vi "Autonomous Independent.vi"() -> ()   [LabVIEW 2018]
doc: "This VI is called when autonomous begins, and will automatically be terminated when autonomous ends. You can carry out timed or sensor driven robot movement independently without needing to return to the caller."
uses:
  <vilib>/Rock Robotics/WPI/Utilities/WPI_GetSetVariantRefNum.vi
  <vilib>/Rock Robotics/Network Tables/NT Read String.vi
  <vilib>/Rock Robotics/Network Tables/NT Write Numeric Array.vi
  <vilib>/Rock Robotics/Network Tables/NT Read Boolean.vi
  <vilib>/Rock Robotics/Network Tables/NT Write Boolean Array.vi
  <vilib>/Rock Robotics/Network Tables/NT Write Boolean.vi
  <vilib>/Rock Robotics/Network Tables/NT Write Number.vi
  <vilib>/Rock Robotics/Network Tables/NT Read Number.vi
  <vilib>/Rock Robotics/Network Tables/NT Read Numeric Array.vi
panel:
  in  "Motor Stall":dbl format="%#_13g"
  out "Current Movement, for debugging":T1 {"Y Joystick Value" scale=1.0..-1.0; "X Joystick Value" scale=-1.0..1.0}
  in  "Array of robot movements":T2(array[cluster])=[{"X Joystick Value"=0.39393939393939403, "Y Joystick Value"=0.0, "Delay (sec)"=1.0, "Movement Name"="turn"}, {"X Joystick Value"=-0.3737373737373737, "Y Joystick Value"=0.0, "Delay (sec)"=1.0, "Movement Name"="turn back"}] {"Y Joystick Value" scale=1.0..-1.0; "X Joystick Value" scale=-1.0..1.0}
  # "Be sure to right-click and choose Data Operations>>Make Current Value default if you want to save the array values with the VI"
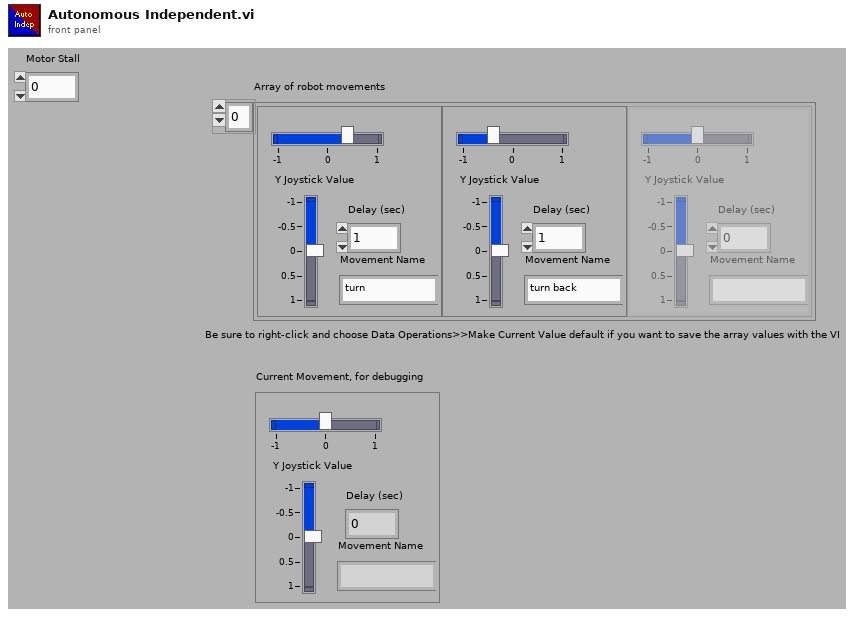
[diagram p1: front panel]
types:
  T1 = cluster{"X Joystick Value":dbl, "Y Joystick Value":dbl, "Delay (sec)":dbl, "Movement Name":string}
  T2 = cluster{"X Joystick Value":dbl, "Y Joystick Value":dbl, "Delay (sec)":dbl, "Movement Name":string}[]
  T3 = typedef "WPI_JoystickDevRef.ctl" = cluster{"Device":T4}
  T4 = typedef "WPI_JoystickDeviceEnum.ctl" = enum16{"USB 0", "USB 1", "USB 2", "USB 3", "USB 4", "USB 5"}
  T5 = typedef "WPI_MotorControlDeviceRef.ctl" = cluster{"DeviceStatus":errorcluster, "Type":T6, "PWM":cluster{"PWM Channel":T7, "DeadBand":T8}, "CAN":cluster{"Device Number":u8, "SetOutput VI Ref":variant, "GetOutput VI Ref":variant, "Enable VI Ref":variant, "Disable VI Ref":variant, "Data":variant}, "Invert":bool, "DIO PWM":cluster{"PWM \"Enable\" Channel":T7, "DIOChannel":T9, "PWM Rate":dbl}}
  T6 = typedef "WPI_MotorControlType.ctl" = enum16{"PWM", "CAN", "DIO PWM"}
  T7 = typedef "FPGA_DIOPWMChannel.ctl" = enum8{"PWM 0", "PWM 1", "PWM 2", "PWM 3", "PWM 4", "PWM 5", "PWM 6", "PWM 7", "PWM 8", "PWM 9", "PWM MXP 0", "PWM MXP 1", "PWM MXP 2", "PWM MXP 3", "PWM MXP 4", "PWM MXP 5", "PWM MXP 6", "PWM MXP 7", "PWM MXP 8", "PWM MXP 9", "Invalid"}
  T8 = typedef "WPI_PWMDeadband.ctl" = cluster{"Name":string, "maxPositivePwm":i32, "minPositivePwm":i32, "centerPwm":i32, "maxNegativePwm":i32, "minNegativePwm":i32, "angularRange":u16}
  T9 = typedef "FPGA_DIOChannel.ctl" = enum8{"DIO 0", "DIO 1", "DIO 2", "DIO 3", "DIO 4", "DIO 5", "DIO 6", "DIO 7", "DIO 8", "DIO 9", "DIO MXP 0", "DIO MXP 1", "DIO MXP 2", "DIO MXP 3", "DIO MXP 4", "DIO MXP 5", "DIO MXP 6", "DIO MXP 7", "DIO MXP 8", "DIO MXP 9", "DIO MXP 10", "DIO MXP 11", "DIO MXP 12", "DIO MXP 13", "DIO MXP 14", "DIO MXP 15", "SPI Port CS1", "SPI Port CS2", "SPI Port CS3", "SPI Port MISO", "SPI Port MOSI", "Invalid"}
  T10 = typedef "WPI_RobotDriveDevRef.ctl" = cluster{"DevStatus":errorcluster, "Motors[]":T5[], "Square Inputs":bool, "Max Output":dbl}
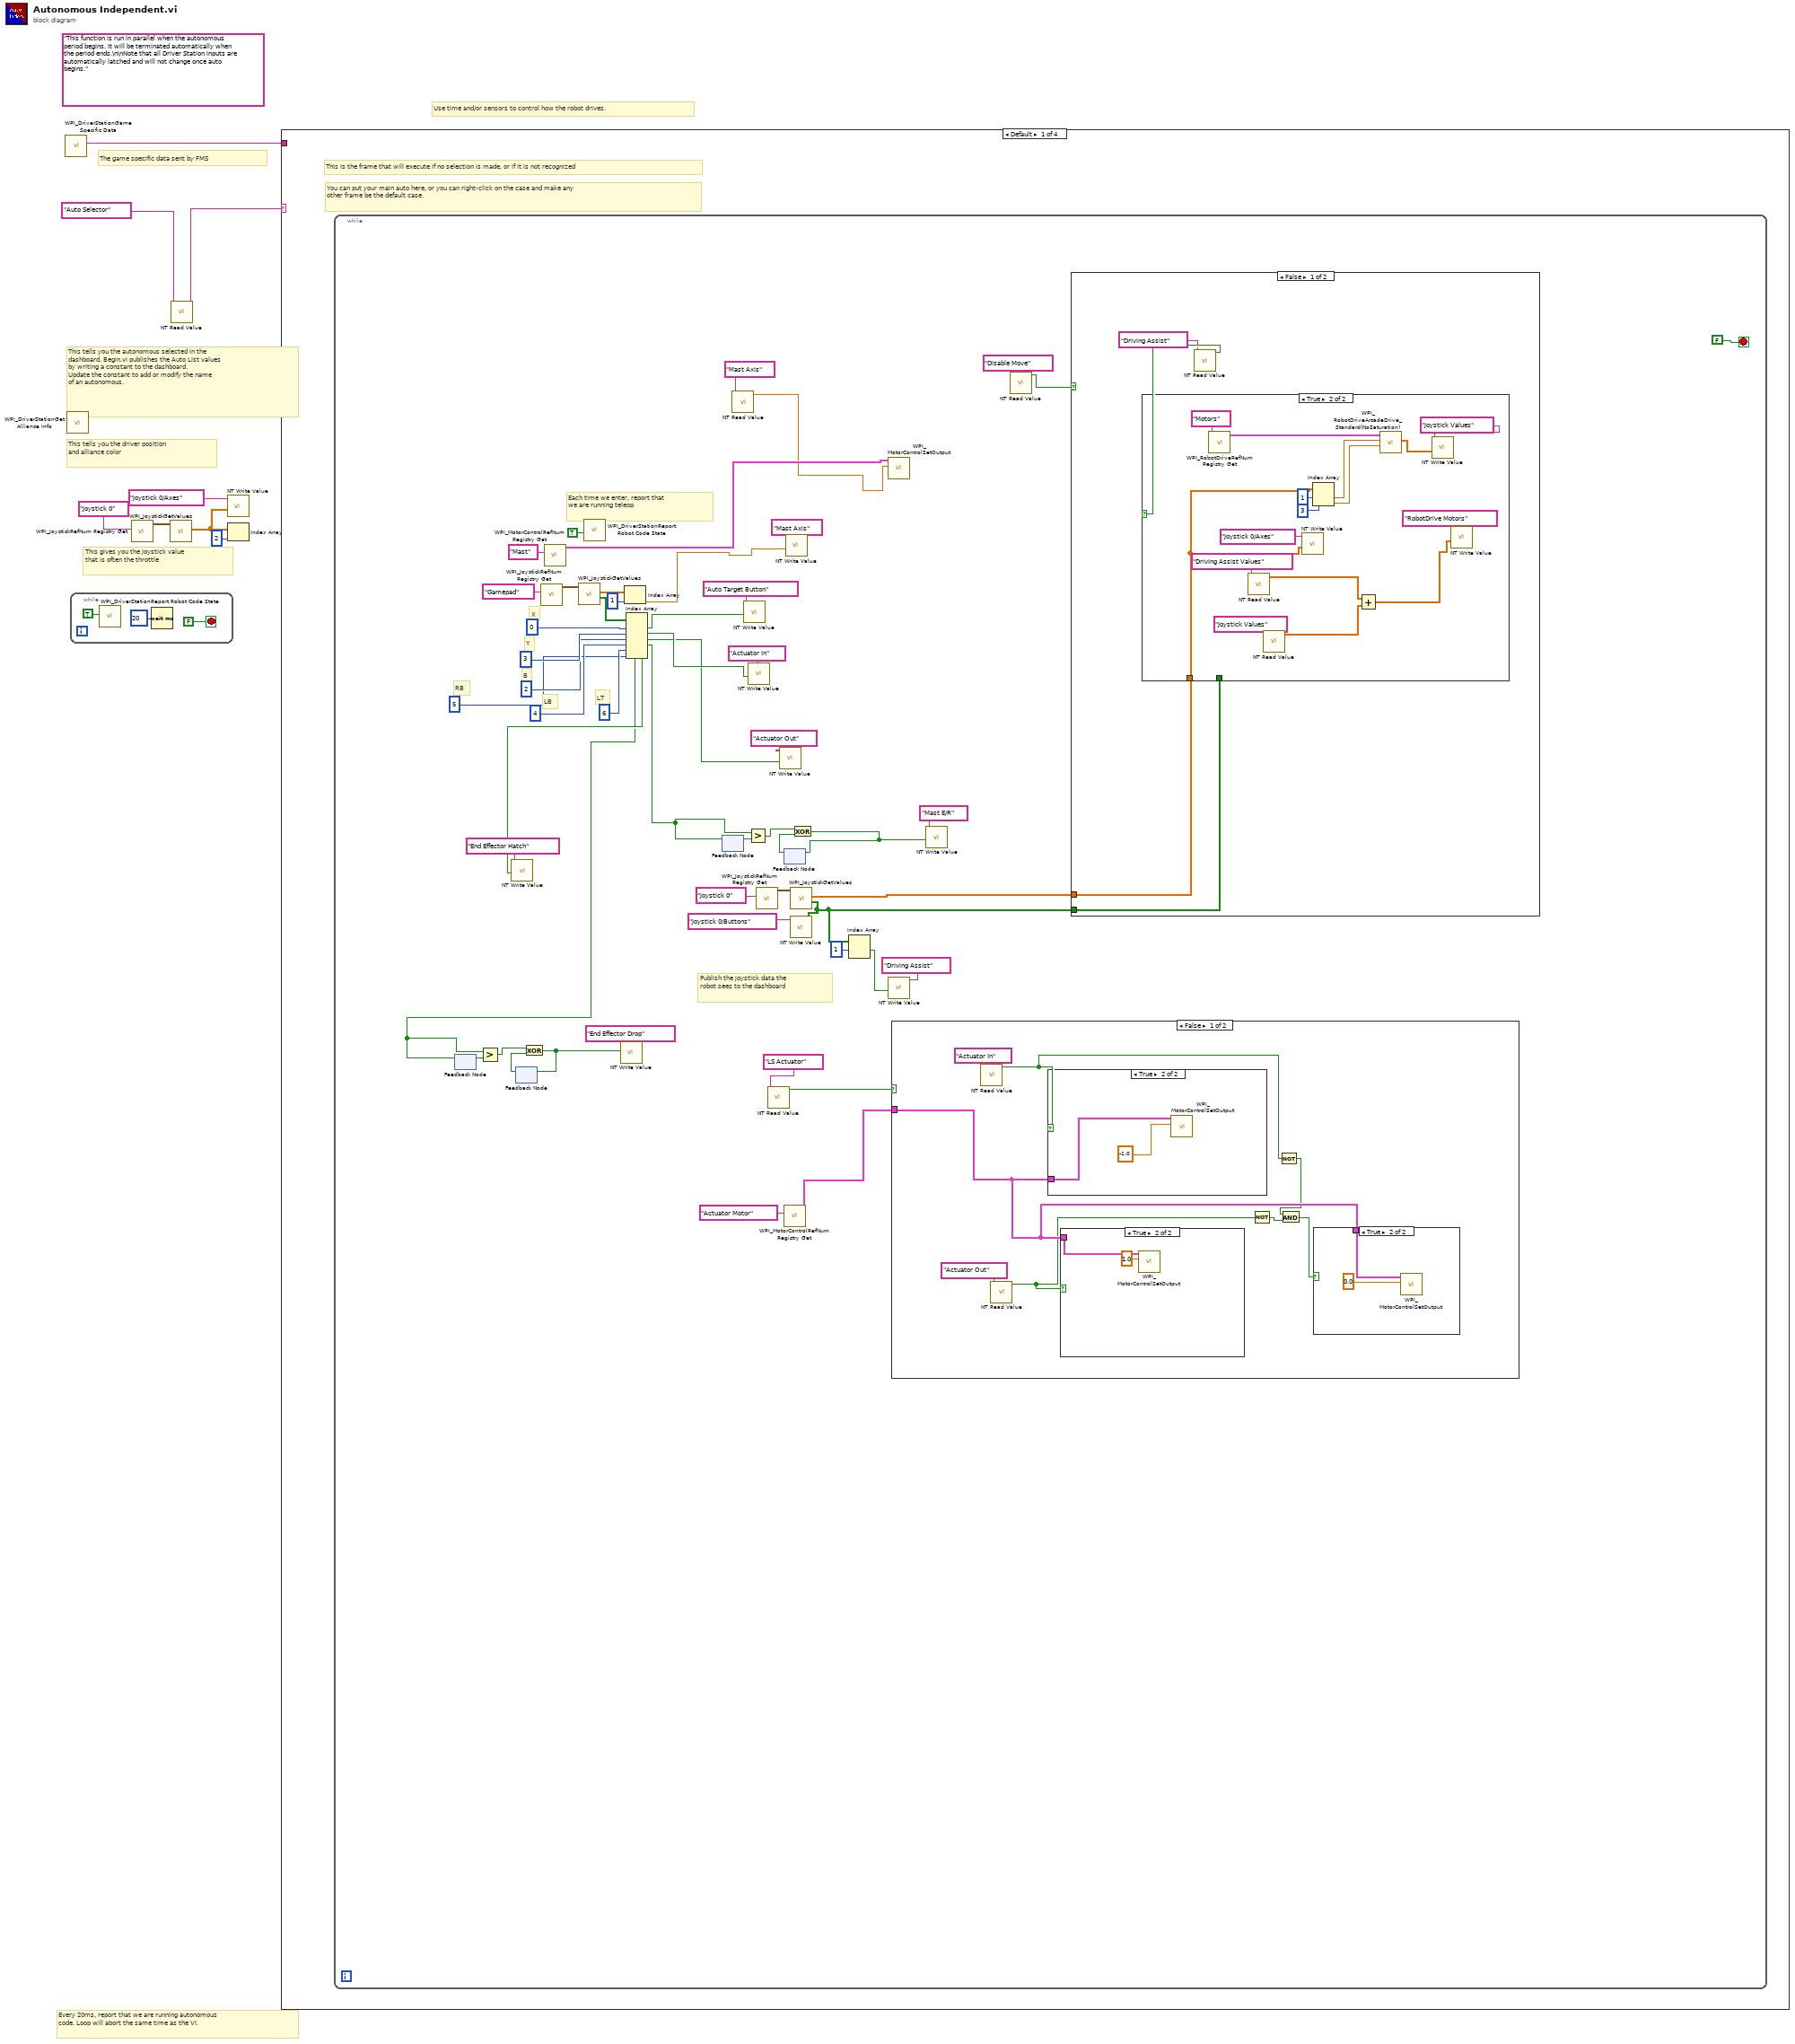
[diagram p0: block diagram]
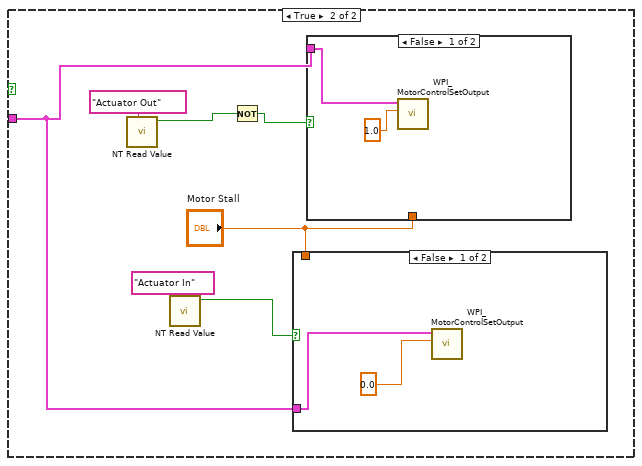
[diagram p5: hidden frame]
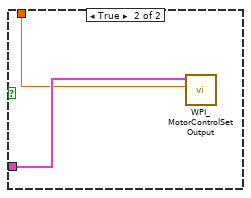
[diagram p6: hidden frame]
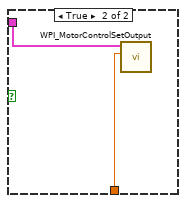
[diagram p7: hidden frame]
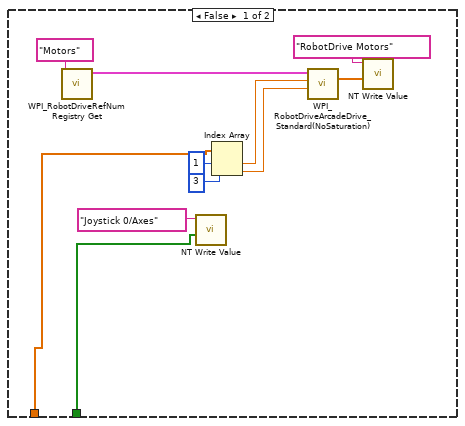
[diagram p8: hidden frame]
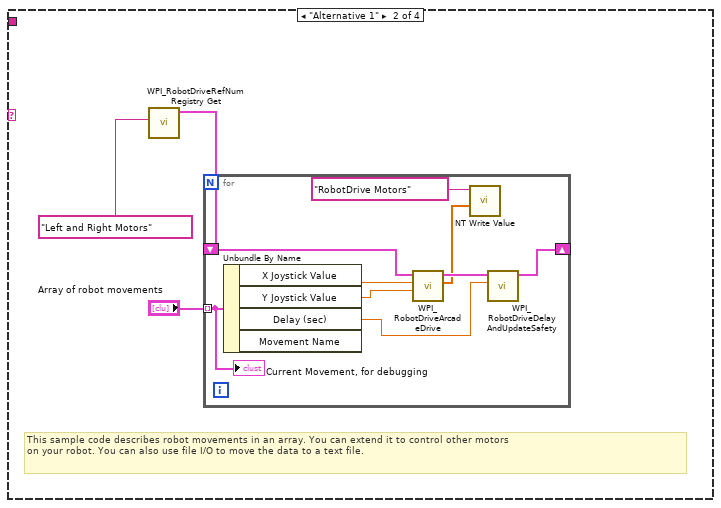
[diagram p10: hidden frame]
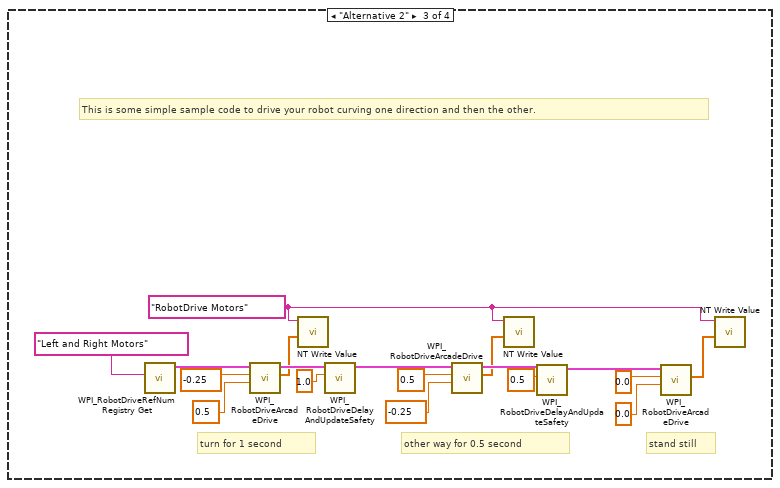
[diagram p11: hidden frame]
diagram:
  (unwired) "This function is run in parallel when the autonomous period begins. It will be terminated automatically when the period ends.\n\nNote that all Driver Station inputs are automatically latched and will not change once auto begins."
  # "The game specific data sent by FMS"
  # "This tells you the autonomous selected in the \ndashboard. Begin.vi publishes the Auto List values\nby writing a constant to the dashboard.\nUpdate the constant to add or modify the name\nof an autonomous."
  # "Every 20ms, report that we are running autonomous\ncode. Loop will abort the same time as the VI."
  # "This gives you the joystick value\nthat is often the throttle"
  # "Use time and/or sensors to control how the robot drives."
  # "This tells you the driver position\nand alliance color"
  n1 = call <vilib>:"WPI_DriverStationGame Specific Data.vi"() -> ("Game Specific Data"=w1:string)  [unwired: 11 in]
  n2 = call <vilib>:"WPI_DriverStationGet Alliance Info.vi"() -> ()  [unwired: 12 out]
  n3 = while {
    stop <- FALSE stop-if-true
    n4 = call <vilib>:"WPI_DriverStationReport Robot Code State.vi"("Autonomous"=TRUE) -> ()  [unwired: 10 in, 1 out]
    n5 = Wait (ms)(milliseconds to wait=u32 20) -> ()  [unwired: 1 out]
  }
  n6 = call <vilib>:"WPI_JoystickRefNum Registry Get.vi"("refnum name"="Joystick 0") -> ("JoystickDevRef"=w7:T3)  [unwired: 1 in, 9 out]
  n7 = call <vilib>:"WPI_JoystickGetValues.vi"("JoystickDevRef"=w7) -> ("Axes"=w3:dbl[])  [unwired: 6 in, 4 out]
  n8 = call-poly <vilib>:"NT Read Value.vi"("Name"="Auto Selector") -> ("String"=w4:string)  [unwired: 9 in, 1 out]
  n9 = call-poly <vilib>:"NT Write Value.vi"("Numeric Array"=w3, "Name"="Joystick 0/Axes") -> ()  [unwired: 9 in, 1 out]
  n10 = Index Array(array=w3, index=2) -> ()  [unwired: 1 out]
  n11 = case shown="Default" w4 {
    tunnel: w1 -> [_ _ _ _]
    frame Default {
      # "You can put your main auto here, or you can right-click on the case and make any\nother frame be the default case."
      # "This is the frame that will execute if no selection is made, or if it is not recognized"
      n12 = while {
        stop <- FALSE stop-if-true
        # "RB"
        # "LT"
        # "LB"
        # "Publish the joystick data the\nrobot sees to the dashboard"
        # "B"
        # "X"
        # "Y"
        # "Each time we enter, report that\nwe are running teleop"
        n13 = feedback #1() -> (w16:bool)  [unwired: 1 in]
        n14 = feedback #2() -> (w14:bool)  [unwired: 1 in]
        n15 = call <vilib>:"WPI_JoystickRefNum Registry Get.vi"("refnum name"="Gamepad") -> ("JoystickDevRef"=w60:T3)  [unwired: 9 in, 1 out]
        n16 = call <vilib>:"WPI_MotorControlRefNum Registry Get.vi"("refnum name"="Mast") -> ("MotorControlDevRef"=w23:T5)  [unwired: 9 in, 1 out]
        n17 = call <vilib>:"WPI_JoystickGetValues.vi"("JoystickDevRef"=w60) -> ("Buttons"=w55:bool[], "Axes"=w59:dbl[])  [unwired: 6 in, 3 out]
        n18 = call <vilib>:"WPI_DriverStationReport Robot Code State.vi"("TeleOp"=TRUE ("Autonomous")) -> ()  [unwired: 10 in, 1 out]
        n19 = Index Array(array=w59, index=1) -> (element=w26:dbl)
        n20 = Index Array(array=w55, index #1=0 ("index"), index #2=3 ("index"), index #3=2 ("index"), index #4=4 ("index"), index #5=6 ("index"), index #6=5 ("index")) -> (element #1=w53:bool, element #2=w47:bool, element #3=w44:bool, element #4=w21:bool, element #5=w13:bool, element #6=w31:bool)
        n21 = feedback-in #1(w13) -> ()
        n22 = Greater?(x=w13, y=w16) -> (0:w15:bool)
        n23 = call-poly <vilib>:"NT Write Value.vi"("Boolean"=w31, "Name"="End Effector Hatch") -> ()  [unwired: 9 in, 1 out]
        n24 = Exclusive Or(1:w14, 2:w15) -> (0:w12:bool)
        n25 = feedback-in #2(w12) -> ()
        n26 = call-poly <vilib>:"NT Write Value.vi"("Boolean"=w12, "Name"="End Effector Drop") -> ()  [unwired: 9 in, 1 out]
        n27 = feedback #3() -> (w20:bool)  [unwired: 1 in]
        n28 = feedback-in #3(w21) -> ()
        n29 = call-poly <vilib>:"NT Read Value.vi"("Name"="Mast Axis") -> ("Numeric"=w22:dbl)  [unwired: 9 in, 1 out]
        n30 = call-poly <vilib>:"NT Write Value.vi"("Boolean"=w53, "Name"="Auto Target Button") -> ()  [unwired: 9 in, 1 out]
        n31 = Greater?(x=w21, y=w20) -> (0:w19:bool)
        n32 = call-poly <vilib>:"NT Write Value.vi"("Boolean"=w47, "Name"="Actuator In") -> ()  [unwired: 9 in, 1 out]
        n33 = call <vilib>:"WPI_JoystickRefNum Registry Get.vi"("refnum name"="Joystick 0") -> ("JoystickDevRef"=w41:T3)  [unwired: 1 in, 9 out]
        n34 = call-poly <vilib>:"NT Read Value.vi"("Name"="LS Actuator") -> ("Boolean"=w50:bool)  [unwired: 9 in, 1 out]
        n35 = call-poly <vilib>:"NT Write Value.vi"("Boolean"=w44, "Name"="Actuator Out") -> ()  [unwired: 9 in, 1 out]
        n36 = feedback #4() -> (w17:bool)  [unwired: 1 in]
        n37 = call <vilib>:"WPI_MotorControlRefNum Registry Get.vi"("refnum name"="Actuator Motor") -> ("MotorControlDevRef"=w42:T5)  [unwired: 9 in, 1 out]
        n38 = call-poly <vilib>:"NT Write Value.vi"("Numeric"=w26, "Name"="Mast Axis") -> ()  [unwired: 9 in, 1 out]
        n39 = call <vilib>:"WPI_JoystickGetValues.vi"("JoystickDevRef"=w41) -> ("Buttons"=w37:bool[], "Axes"=w39:dbl[])  [unwired: 6 in, 3 out]
        n40 = call-poly <vilib>:"NT Write Value.vi"("Boolean Array"=w37, "Name"="Joystick 0/Buttons") -> ()  [unwired: 9 in, 1 out]
        n41 = Exclusive Or(1:w17, 2:w19) -> (0:w18:bool)
        n42 = feedback-in #4(w18) -> ()
        n43 = Index Array(array=w37, index #1=1 ("index")) -> (element #1=w35:bool)  [unwired: 1 in, 1 out]
        n44 = call <vilib>:"WPI_MotorControlSetOutput.vi"("Output"=w22, "MotorControlDevRef"=w23) -> ()  [unwired: 7 in, 3 out]
        n45 = call-poly <vilib>:"NT Write Value.vi"("Boolean"=w35, "Name"="Driving Assist") -> ()  [unwired: 9 in, 1 out]
        n46 = case shown="False" w50 {
          tunnel: w42 -> [w69 w80]
          frame False {
            n47 = call-poly <vilib>:"NT Read Value.vi"("Name"="Actuator In") -> ("Boolean"=w66:bool)  [unwired: 9 in, 1 out]
            n48 = call-poly <vilib>:"NT Read Value.vi"("Name"="Actuator Out") -> ("Boolean"=w67:bool)  [unwired: 9 in, 1 out]
            n49 = case shown="True" w66 {
              tunnel: w69 -> [_ w77]
              frame False {
              }
              frame True {
                n50 = call <vilib>:"WPI_MotorControlSetOutput.vi"("Output"=-1.0, "MotorControlDevRef"=w77) -> ()  [unwired: 7 in, 3 out]
              }
            }
            n51 = case shown="True" w67 {
              tunnel: w69 -> [_ w76]
              frame False {
              }
              frame True {
                n52 = call <vilib>:"WPI_MotorControlSetOutput.vi"("Output"=1.0, "MotorControlDevRef"=w76) -> ()  [unwired: 7 in, 3 out]
              }
            }
            n53 = Not(x=w67) -> (.not. x?=w68:bool)
            n54 = Not(x=w66) -> (.not. x?=w65:bool)
            n55 = And(x=w65, y=w68) -> (x .and. y?=w70:bool)
            n56 = case shown="True" w70 {
              tunnel: w69 -> [_ w73]
              frame False {
              }
              frame True {
                n57 = call <vilib>:"WPI_MotorControlSetOutput.vi"("Output"=0.0, "MotorControlDevRef"=w73) -> ()  [unwired: 7 in, 3 out]
              }
            }
          }
          frame True {
            n58 = call-poly <vilib>:"NT Read Value.vi"("Name"="Actuator Out") -> ("Boolean"=w84:bool)  [unwired: 9 in, 1 out]
            n59 = call-poly <vilib>:"NT Read Value.vi"("Name"="Actuator In") -> ("Boolean"=w81:bool)  [unwired: 9 in, 1 out]
            n60 = Not(x=w84) -> (.not. x?=w83:bool)
            n61 = case shown="False" w81 {
              tunnel: w80 -> [w86 w89]
              tunnel: "Motor Stall" -> [_ w88]
              frame False {
                n62 = call <vilib>:"WPI_MotorControlSetOutput.vi"("Output"=0.0, "MotorControlDevRef"=w86) -> ()  [unwired: 7 in, 3 out]
              }
              frame True {
                n63 = call <vilib>:"WPI_MotorControlSetOutput.vi"("Output"=w88, "MotorControlDevRef"=w89) -> ()  [unwired: 7 in, 3 out]
              }
            }
            n64 = case shown="False" w83 {
              tunnel: w80 -> [w91 w93]
              tunnel: "Motor Stall" -> [_ w92]
              frame False {
                n65 = call <vilib>:"WPI_MotorControlSetOutput.vi"("Output"=1.0, "MotorControlDevRef"=w91) -> ()  [unwired: 7 in, 3 out]
              }
              frame True {
                n66 = call <vilib>:"WPI_MotorControlSetOutput.vi"("Output"=w92, "MotorControlDevRef"=w93) -> ()  [unwired: 7 in, 3 out]
              }
            }
          }
        }
        n67 = call-poly <vilib>:"NT Write Value.vi"("Boolean"=w18, "Name"="Mast E/R") -> ()  [unwired: 9 in, 1 out]
        n68 = call-poly <vilib>:"NT Read Value.vi"("Name"="Disable Move") -> ("Boolean"=w57:bool)  [unwired: 9 in, 1 out]
        n69 = case shown="False" w57 {
          tunnel: w37 -> [w96 _]
          tunnel: w39 -> [w97 _]
          frame False {
            n70 = call-poly <vilib>:"NT Read Value.vi"("Name"="Driving Assist") -> ("Boolean"=w95:bool)  [unwired: 9 in, 1 out]
            n71 = case shown="True" w95 {
              tunnel: w97 -> [w99 w117]
              tunnel: w96 -> [w98 _]
              frame False {
                n72 = call <vilib>:"WPI_RobotDriveRefNum Registry Get.vi"("refnum name"="Motors") -> ("RobotDriveDevRef"=w107:T10)  [unwired: 1 in, 9 out]
                n73 = call-poly <vilib>:"NT Write Value.vi"("Boolean Array"=w98, "Name"="Joystick 0/Axes") -> ()  [unwired: 9 in, 1 out]
                n74 = Index Array(array=w99, index #1=1 ("index"), index #2=3 ("index")) -> (element #1=w106:dbl, element #2=w105:dbl)
                n75 = call <vilib>:"WPI_RobotDriveArcadeDrive_Standard(NoSaturation).vi"("Y axis value"=w105, "X axis value"=w106, "RobotDriveDevRef"=w107) -> ("Motor Values"=w103:dbl[])  [unwired: 1 in, 7 out]
                n76 = call-poly <vilib>:"NT Write Value.vi"("Numeric Array"=w103, "Name"="RobotDrive Motors") -> ()  [unwired: 9 in, 1 out]
              }
              frame True {
                n77 = call <vilib>:"WPI_RobotDriveRefNum Registry Get.vi"("refnum name"="Motors") -> ("RobotDriveDevRef"=w123:T10)  [unwired: 1 in, 9 out]
                n78 = call-poly <vilib>:"NT Read Value.vi"("Name"="Driving Assist Values") -> ("Numeric Array"=w112:dbl[])  [unwired: 9 in, 1 out]
                n79 = call-poly <vilib>:"NT Read Value.vi"("Name"="Joystick Values") -> ("Numeric Array"=w111:dbl[])  [unwired: 9 in, 1 out]
                n80 = call-poly <vilib>:"NT Write Value.vi"("Numeric Array"=w117, "Name"="Joystick 0/Axes") -> ()  [unwired: 9 in, 1 out]
                n81 = Index Array(array=w117, index #1=1 ("index"), index #2=3 ("index")) -> (element #1=w122:dbl, element #2=w121:dbl)
                n82 = Add(x=w112, y=w111) -> (x+y=w109:dbl[])
                n83 = call <vilib>:"WPI_RobotDriveArcadeDrive_Standard(NoSaturation).vi"("Y axis value"=w121, "X axis value"=w122, "RobotDriveDevRef"=w123) -> ("Motor Values"=w115:dbl[])  [unwired: 1 in, 7 out]
                n84 = call-poly <vilib>:"NT Write Value.vi"("Numeric Array"=w115, "Name"="Joystick Values") -> ()  [unwired: 9 in, 1 out]
                n85 = call-poly <vilib>:"NT Write Value.vi"("Numeric Array"=w109, "Name"="RobotDrive Motors") -> ()  [unwired: 9 in, 1 out]
              }
            }
          }
          frame True {
          }
        }
      }
    }
    frame "Alternative 1" {
      # "This sample code describes robot movements in an array. You can extend it to control other motors\non your robot. You can also use file I/O to move the data to a text file."
      n86 = call <vilib>:"WPI_RobotDriveRefNum Registry Get.vi"("refnum name"="Left and Right Motors") -> ("RobotDriveDevRef"=w126:T10)  [unwired: 1 in, 9 out]
      n87 = for {
        shift-right: [w134] -> _
        shift-left: w126 -> [w135]
        tunnel: "Array of robot movements" -> [w130] mode=indexing
        n88 = Unbundle By Name(w130) -> ("X Joystick Value"=w133:dbl, "Y Joystick Value"=w132:dbl, "Delay (sec)"=w131:dbl)  [unwired: 1 out]
        n89 = call-poly <vilib>:"WPI_RobotDriveArcadeDrive.vi"("Y axis value"=w132, "X axis value"=w133, "RobotDriveDevRef"=w135) -> ("Motor Values"=w128:dbl[], "RobotDriveDevRef"=w136:T10)  [unwired: 1 in, 6 out]
        n90 = call-poly <vilib>:"NT Write Value.vi"("Numeric Array"=w128, "Name"="RobotDrive Motors") -> ()  [unwired: 9 in, 1 out]
        n91 = call <vilib>:"WPI_RobotDriveDelayAndUpdateSafety.vi"("Delay (s)"=w131, "RobotDriveDevRef"=w136) -> ("RobotDriveDevRef 2"=w134:T10)  [unwired: 8 in, 1 out]
        "Current Movement, for debugging" <- w130
      }
    }
    frame "Alternative 2" {
      w138 = "RobotDrive Motors" ("Name")
      # "This is some simple sample code to drive your robot curving one direction and then the other."
      # "stand still"
      # "other way for 0.5 second"
      # "turn for 1 second"
      n92 = call <vilib>:"WPI_RobotDriveRefNum Registry Get.vi"("refnum name"="Left and Right Motors") -> ("RobotDriveDevRef"=w154:T10)  [unwired: 1 in, 9 out]
      n93 = call-poly <vilib>:"WPI_RobotDriveArcadeDrive.vi"("Y axis value"=0.5 ("X axis value"), "X axis value"=-0.25, "RobotDriveDevRef"=w154) -> ("Motor Values"=w137:dbl[], "RobotDriveDevRef"=w147:T10)  [unwired: 1 in, 6 out]
      n94 = call-poly <vilib>:"NT Write Value.vi"("Numeric Array"=w137, "Name"=w138) -> ()  [unwired: 9 in, 1 out]
      n95 = call <vilib>:"WPI_RobotDriveDelayAndUpdateSafety.vi"("Delay (s)"=1.0, "RobotDriveDevRef"=w147) -> ("RobotDriveDevRef 2"=w148:T10)  [unwired: 8 in, 1 out]
      n96 = call-poly <vilib>:"WPI_RobotDriveArcadeDrive.vi"("Y axis value"=-0.25 ("X axis value"), "X axis value"=0.5, "RobotDriveDevRef"=w148) -> ("Motor Values"=w139:dbl[], "RobotDriveDevRef"=w149:T10)  [unwired: 1 in, 6 out]
      n97 = call-poly <vilib>:"NT Write Value.vi"("Numeric Array"=w139, "Name"=w138) -> ()  [unwired: 9 in, 1 out]
      n98 = call <vilib>:"WPI_RobotDriveDelayAndUpdateSafety.vi"("Delay (s)"=0.5, "RobotDriveDevRef"=w149) -> ("RobotDriveDevRef 2"=w150:T10)  [unwired: 8 in, 1 out]
      n99 = call-poly <vilib>:"WPI_RobotDriveArcadeDrive.vi"("Y axis value"=0.0 ("X axis value"), "X axis value"=0.0, "RobotDriveDevRef"=w150) -> ("Motor Values"=w140:dbl[])  [unwired: 1 in, 7 out]
      n100 = call-poly <vilib>:"NT Write Value.vi"("Numeric Array"=w140, "Name"=w138) -> ()  [unwired: 9 in, 1 out]
    }
    frame "Your Turn" {
    }
  }
